vi "8bitTo16bit.vi"(1 "input_byte":u8[](array[numeric])) -> (0 "output_int16":i32[](array[numeric]))   [LabVIEW 2013]
panel:
  out "msb":u8
  out "lsb":u8
  # "The input of this VI is a byte vector of 8 indexes, that contains 4 uint16_t separeted into 2 bytes in the vector.\nEach two bytes represent a number os 16 bits, where the fist bite is the LSB and the second ins MSB"
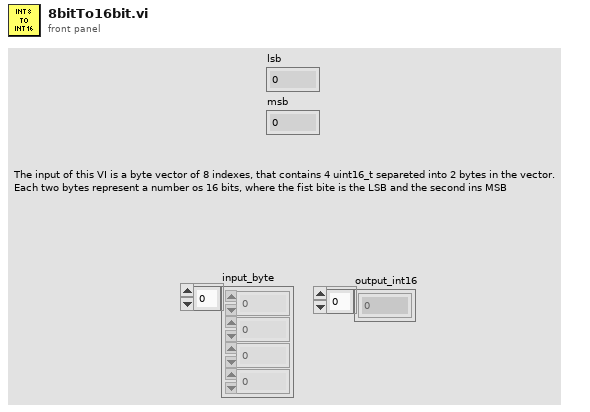
[diagram p1: front panel]
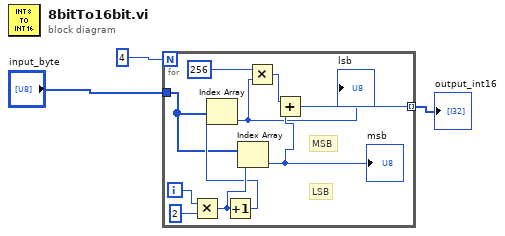
[diagram p0: block diagram]
diagram:
  n1 = for {
    N: 4 -> [_]
    tunnel: "input_byte" -> [w6]
    tunnel: [w9] -> w2 mode=indexing
    i -> [w13]
    # "LSB"
    # "MSB"
    n2 = Multiply(x=w13, y=2) -> (x*y=w8:i32)
    n3 = Increment(x=w8) -> (x+1=w7:i32)
    n4 = Index Array(array=w6, index=w7) -> (element=w4:u8)
    "lsb" <- w4
    n5 = Index Array(array=w6, index=w8) -> (element=w5:u8)
    "msb" <- w5
    n6 = Multiply(x=256, y=w4) -> (x*y=w10:i32)
    n7 = Add(x=w10, y=w5) -> (x+y=w9:i32)
  }
  "output_int16" <- w2
